vi "cluster_unbundle_bundle_example1.vi"() -> ()   [LabVIEW 2020]
panel:
  out "true":bool
  in  "message":string
  out "age 3":dbl
  in  "age":dbl
  in  "Cluster":cluster{"salary":dbl, "name":string, "age":dbl}
  out "age 2":dbl
  out "name 2":string
  out "salary 2":dbl
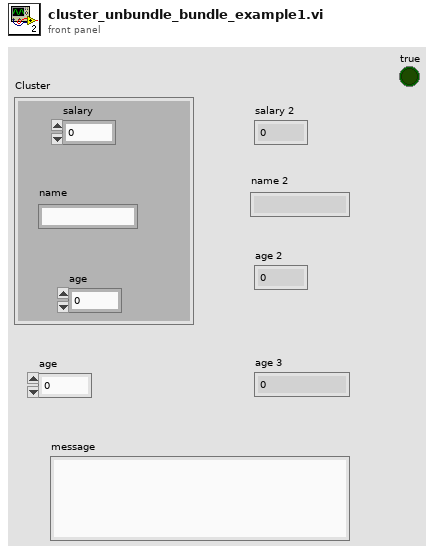
[diagram p1: front panel]
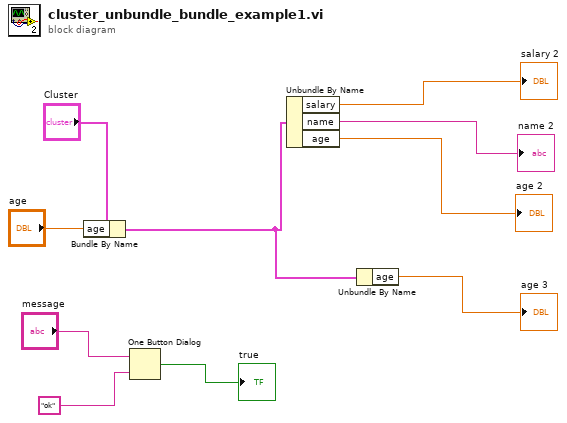
[diagram p0: block diagram]
diagram:
  n1 = Bundle By Name "Bundle By Name"(cluster="Cluster", "age"="age") -> (w5:cluster{"salary":dbl, "name":string, "age":dbl})
  n2 = One Button Dialog(message="message", button name ("OK")="ok") -> (true=→"true":bool)
  n3 = Unbundle By Name "Unbundle By Name"(w5) -> ("salary"=→"salary 2":dbl, "name"=→"name 2":string, "age"=→"age 2":dbl)
  n4 = Unbundle By Name "Unbundle By Name"(w5) -> ("age"=→"age 3":dbl)
